vi "initialise.vi"(8 "error in (no error)":errorcluster, 11 "DL090216RangeOffsetImageProcessor in":refnum<class "ImageProcessorDL090216RangeOffset.lvclass">) -> (0 "error out":errorcluster, 3 "DL090216RangeOffsetImageProcessor out":refnum<class "ImageProcessorDL090216RangeOffset.lvclass">)   [LabVIEW 2010, in "ImageProcessorDL090216RangeOffset.lvclass"]
uses:
  ImageProcessorDL090216RangeOffset.lvclass
  GenericImageProcessor/GenericImageProcessor/GenericImageProcessor.lvclass
  common/clusters/range_offset_cluster.ctl
  ImageProcessorDL090216RangeOffset.lvclass/ImageProcessorDL090216RangeOffset.ctl
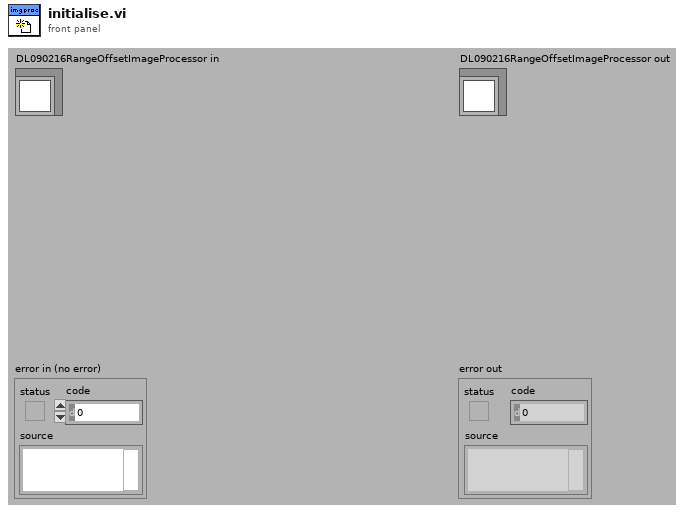
[diagram p1: front panel]
types:
  T1 = typedef "range_offset_cluster.ctl" = cluster{"range":dbl, "offset":dbl}
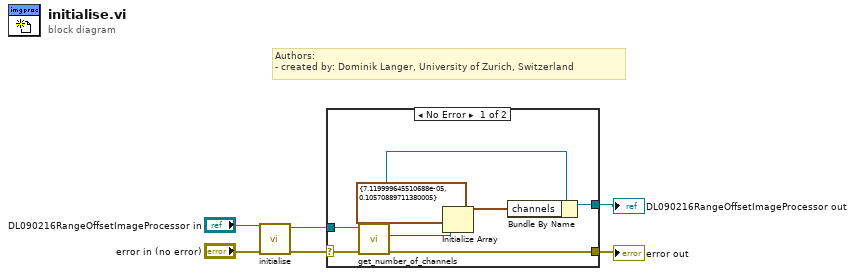
[diagram p0: block diagram]
diagram:
  # "Authors: \n- created by: Dominik Langer, University of Zurich, Switzerland"
  n1 = call-parent "initialise.vi"("error in (no error)"="error in (no error)", "GenericImageProcessor in"="DL090216RangeOffsetImageProcessor in") -> ("error out"=w1:errorcluster, "GenericImageProcessor out"=w3:refnum<class "ImageProcessorDL090216RangeOffset.lvclass">)  [unwired: 8 out]
  n2 = case shown="No Error" w1 {
    selector: w1 -> [w14 w16]
    tunnel: [w13 w16] -> w6
    tunnel: [w10 w15] -> w5
    tunnel: w3 -> [w12 w15]
    frame No Error {
      n3 = call "get_number_of_channels.vi"("error in (no error)"=w14, "GenericImageProcessor.lvclass in"=w12) -> ("error out"=w13:errorcluster, "number of channels"=w8:i32, "GenericImageProcessor.lvclass out"=w11:refnum<class "ImageProcessorDL090216RangeOffset.lvclass">)  [unwired: 7 out]
      n4 = Initialize Array(T1 {"range"=7.119999645510688e-05, "offset"=0.10570889711380005} ("master"), w8) -> (w9:T1[])
      n5 = Bundle By Name(cluster=w11, "channels"=w9) -> (w10:refnum<class "ImageProcessorDL090216RangeOffset.lvclass">)
    }
    frame Error {
    }
  }
  "error out" <- w6
  "DL090216RangeOffsetImageProcessor out" <- w5
